vi "PCA example with Iris Data-set.vi"() -> ()   [LabVIEW 2020]
doc: "Principal Component Analysis applied to the Iris dataset."
uses:
  <vilib>/Math Plots/3D Math Plots/3D Scatter/3D Scatter XCtrl/3D Scatter.xctl
  Model/Unsupervised/Decomposition/PCA/Controls/pca_params.ctl
  <vilib>/Math Plots/3D Math Plots/3D Plot/3D Plot Datatype/3D Plot Datatype.lvclass
  Display/_Controls/Style.ctl
  Model/Unsupervised/Decomposition/PCA/PCA.lvclass
  C:/Users/cipop/TDF Dropbox/2_Technologies de France/1 - Services et Etudes/PLAIY/2 - DEV/PLAIYLAB/code/Model/Model.lvclass
  Model/Unsupervised/Decomposition/PCA/PCA.vi
panel:
  out "error out 2":errorcluster
  in  "error in":errorcluster
  in  "Local":cluster{"X":dbl[][], "y":dbl[]}
  out "3D Scatter":refnum<class "3D Plot Datatype.lvclass">[](xcontrol)
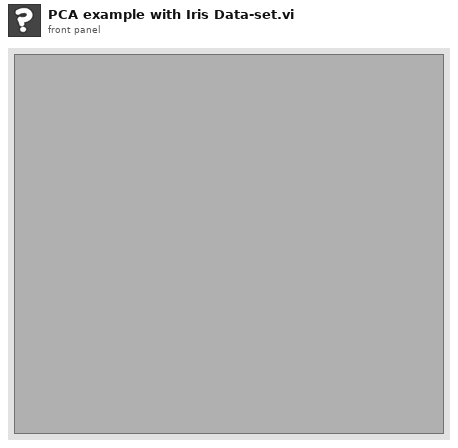
[diagram p1: front panel]
types:
  T1 = cluster{"n_components_type":string, "n_components_int":i32, "n_components_float":dbl}
  T2 = typedef "pca_params.ctl" = cluster{"n_components":cluster{"n_components_type":string, "n_components_int":i32, "n_components_float":dbl}, "copy":bool, "whiten":bool, "svd_solver":string, "tol":dbl, "iterated_power":cluster{"iterated_power_type":string, "iterated_power_int":dbl}, "random_state":dbl}
  T3 = typedef "Style.ctl" = enum16{"Empty circle", "Full circle", "Empty square", "Full square", "Cross"}
  T4 = cluster{"Parameter":cluster{"3D Plot":refnum<class "3D Plot Datatype.lvclass">[], "3D Scatter":refnum<vi>, "Data":cluster{"X":dbl[][], "Predict":dbl[][]}, "Display":cluster{"Choice":enum16{"All", "Train", "Test"}, "Indexe":cluster{"X":i32, "Y":i32, "Z":i32}}, "Point Property":cluster{"Style":T3, "Label Color":u32[]}}}
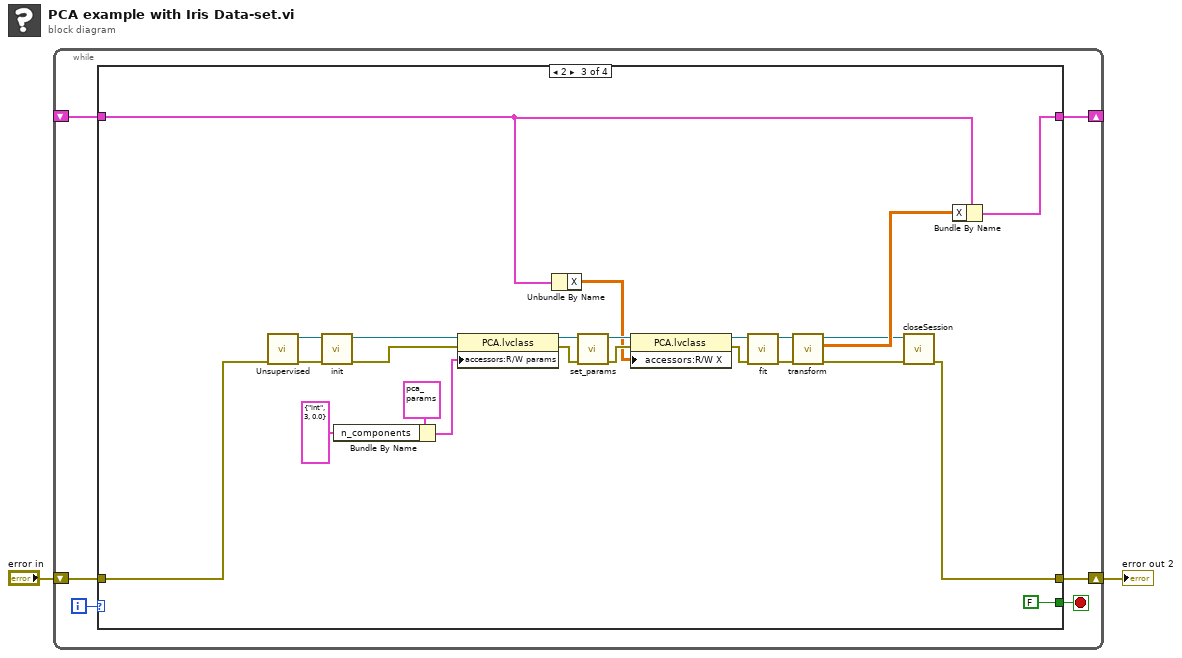
[diagram p0: block diagram]
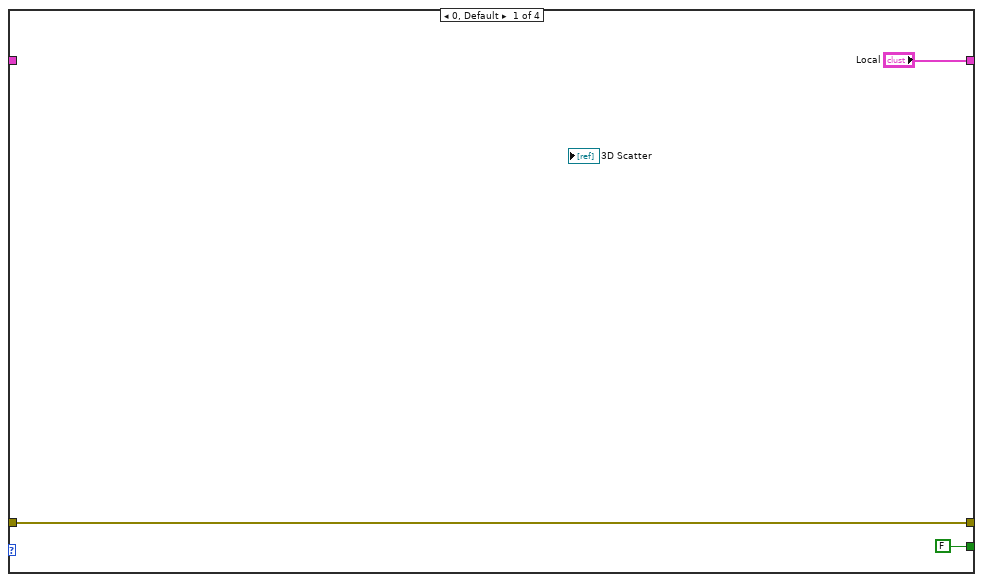
[diagram p2: hidden frame]
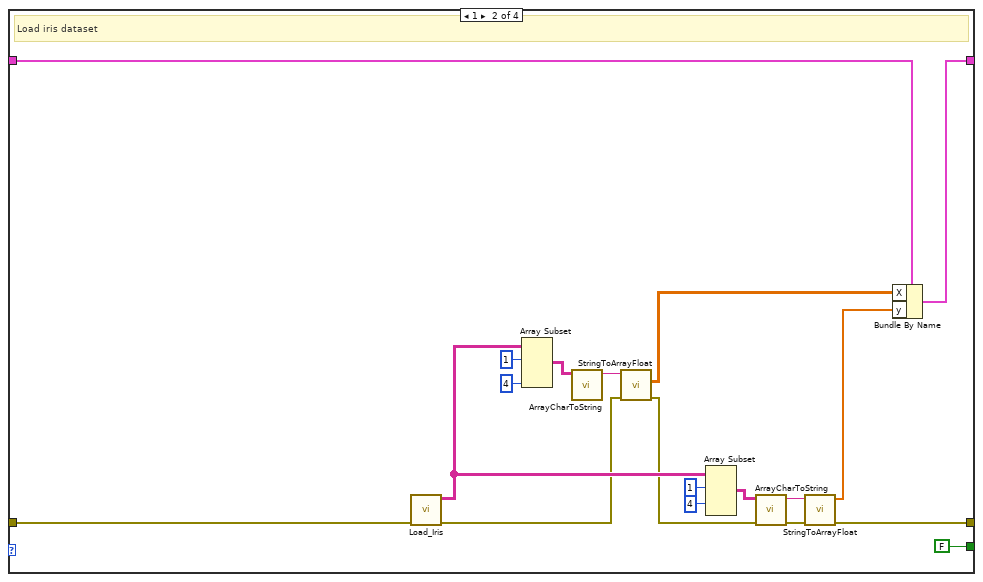
[diagram p3: hidden frame]
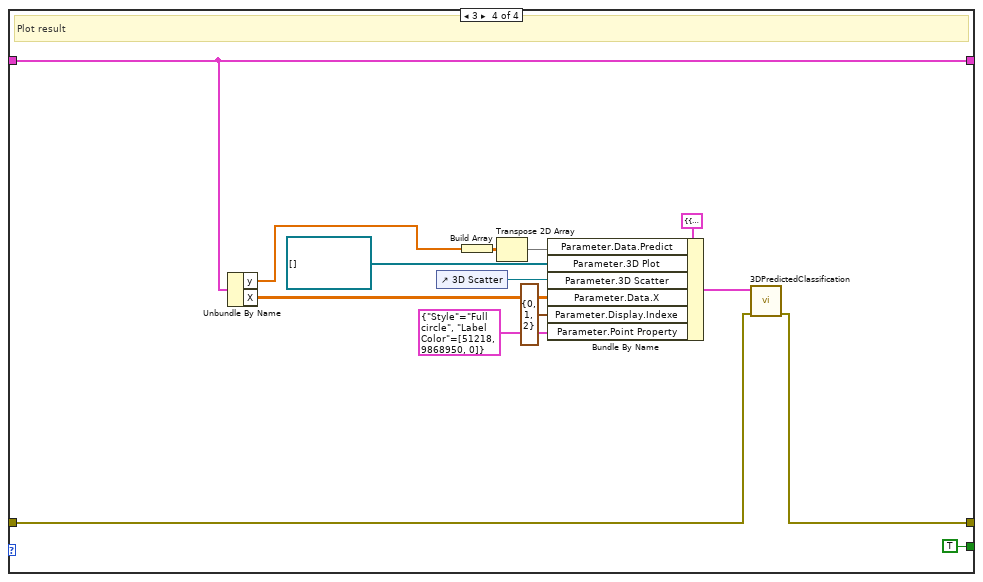
[diagram p4: hidden frame]
diagram:
  n1 = while {
    shift-right: [w6] -> w1
    shift-left: "error in" -> [w7]
    shift-right: [w5] -> _
    shift-left: _ -> [w4]
    i -> [w8]
    stop <- w3 stop-if-true
    n2 = case shown="2" w8 {
      tunnel: w7 -> [w10 w16 w42 w54]
      tunnel: [w10 w13 w40 w62] -> w6
      tunnel: ["Local" w27 w46 w58] -> w5
      tunnel: w4 -> [_ w28 w47 w58]
      tunnel: [FALSE FALSE FALSE TRUE] -> w3
      frame 0, Default {
      }
      frame 1 {
        # "Load iris dataset"
        n3 = call "Load_Iris.vi"("error in"=w16) -> ("error out"=w17:errorcluster, "Tableau"=w22:string[][])  [unwired: 9 in]
        n4 = Array Subset(array=w22, index (row)=1 ("index"), length (col)=4 ("length")) -> (w20:string[][])  [unwired: 2 in]
        n5 = call "ArrayCharToString.vi"("TAB"=w20) -> ("Instruction"=w21:string)  [unwired: 10 in]
        n6 = call "StringToArrayFloat.vi"("entrée d'erreur (pas d'erreur)"=w17, "Return value"=w21) -> ("error IO"=w14:errorcluster, "2DArray"=w15:dbl[][])  [unwired: 7 in, 1 out]
        n7 = Array Subset(array=w22, index (row)=1 ("index"), index (col)=4 ("index")) -> (w18:string[][])  [unwired: 2 in]
        n8 = call "ArrayCharToString.vi"("TAB"=w18) -> ("Instruction"=w19:string)  [unwired: 10 in]
        n9 = call "StringToArrayFloat.vi"("entrée d'erreur (pas d'erreur)"=w14, "Return value"=w19) -> ("error IO"=w13:errorcluster, "1DArray"=w12:dbl[])  [unwired: 7 in, 1 out]
        n10 = Bundle By Name(cluster=w28, "X"=w15, "y"=w12) -> (w27:cluster{"X":dbl[][], "y":dbl[]})
      }
      frame 2 {
        n11 = call-poly "Unsupervised.vi"("error in"=w42) -> ("error out"=w43:errorcluster, "out"=w44:refnum<class "PCA.lvclass">)  [unwired: 9 in]
        n12 = call-dynamic "init.vi"("error in (no error)"=w43, "Model en entrée"=w44) -> ("error out"=w48:errorcluster, "Model en sortie"=w52:refnum<class "PCA.lvclass">)  [unwired: 8 in]
        n13 = Bundle By Name(cluster=T2 {"n_components"={"n_components_type"="int", "n_components_int"=2, "n_components_float"=0.0}, "copy"=TRUE, "whiten"=FALSE, "svd_solver"="auto", "tol"=0.0, "iterated_power"={"iterated_power_type"="auto", "iterated_power_int"=0.0}, "random_state"=0.0} ("R/W params"), "n_components"=T1 {"n_components_type"="int", "n_components_int"=3, "n_components_float"=0.0}) -> (w30:T2)
        n14 = property class="PCA.lvclass"(reference=w52, error in=w48, "accessors:R/W params"=w30) -> (reference out=w51:refnum<class "PCA.lvclass">, error out=w45:errorcluster)
        n15 = Unbundle By Name(w47) -> ("X"=w41:dbl[][])
        n16 = call-dynamic "set_params.vi"("error in (no error)"=w45, "PCA.lvclass 2"=w51) -> ("error out"=w49:errorcluster, "PCA.lvclass"=w50:refnum<class "PCA.lvclass">)  [unwired: 8 in]
        n17 = property class="PCA.lvclass"(reference=w50, error in=w49, "accessors:R/W X"=w41) -> (reference out=w39:refnum<class "PCA.lvclass">, error out=w38:errorcluster)
        n18 = call-dynamic "fit.vi"("error in (no error)"=w38, "Decomposition.lvclass 2"=w39) -> ("error out"=w33:errorcluster, "Decomposition.lvclass"=w34:refnum<class "PCA.lvclass">)  [unwired: 8 in]
        n19 = call-dynamic "transform.vi"("error in (no error)"=w33, "Decomposition.lvclass 2"=w34) -> ("error out"=w35:errorcluster, "X_new"=w37:dbl[][], "Decomposition.lvclass"=w36:refnum<class "PCA.lvclass">)  [unwired: 7 in]
        n20 = call-dynamic "closeSession.vi"("error in"=w35, "Python en entrée"=w36) -> ("error out"=w40:errorcluster)  [unwired: 8 in, 1 out]
        n21 = Bundle By Name(cluster=w47, "X"=w37) -> (w46:cluster{"X":dbl[][], "y":dbl[]})
      }
      frame 3 {
        # "Plot result"
        n22 = Unbundle By Name(w58) -> ("y"=w57:dbl[], "X"=w59:dbl[][])
        n23 = control-ref of="3D Scatter"() -> (w60:refnum<vi>)
        n24 = Build Array(w57) -> (w56:dbl[][])
        n25 = Transpose 2D Array(2D array=w56) -> (transposed array=w55:dbl[][])
        n26 = Bundle By Name(cluster=T4 {"Parameter"={"3D Plot"=[], "3D Scatter"=refnum, "Data"={"X"=[], "Predict"=[]}, "Display"={"Choice"=enum."All", "Indexe"={"X"=0, "Y"=1, "Z"=2}}, "Point Property"={"Style"=enum."Full circle", "Label Color"=[8978528, 4367871, 1985280]}}} ("Parameters"), "Parameter.Data.Predict"=w55, "Parameter.3D Plot"=refnum<class "3D Plot Datatype.lvclass">[] [] ("3D Scatter"), "Parameter.3D Scatter"=w60, "Parameter.Data.X"=w59, "Parameter.Display.Indexe"=cluster{"X":i32, "Y":i32, "Z":i32} {"X"=0, "Y"=1, "Z"=2}, "Parameter.Point Property"=cluster{"Style":T3, "Label Color":u32[]} {"Style"=enum."Full circle", "Label Color"=[51218, 9868950, 0]} ("Point Property")) -> (w67:T4)
        n27 = call "3DPredictedClassification.vi"("error in"=w54, "Parameters"=w67) -> ("error out"=w62:errorcluster)  [unwired: 8 in, 1 out]
      }
    }
  }
  "error out 2" <- w1
